vi "Initialize Debug Attribute.vi"(7 "Attribute.Debug in":refnum<class "Attribute.Debug.lvclass">, 11 "Behavior (Normal)":T1) -> (3 "Attribute.Debug out":refnum<class "Attribute.Debug.lvclass">)   [LabVIEW 2019, in "Debug.lvlib" / "Attribute.Debug.lvclass"]
uses:
  Attribute.Debug.lvclass
  DebugBehavior.ctl
  <vilib>/JKI/JKI SMO/smo.lvlibp/Definitions/def.SMO/Scope -- Enum.ctl
  Attribute.Debug.lvclass/Attribute.Debug.ctl
  <vilib>/JKI/JKI SMO/smo.lvlibp/Support/Attribute/Attribute.lvclass
  <vilib>/JKI/JKI SMO/smo.lvlibp/Definitions/def.SMO/def.SMO.lvclass
  C:/Program Files (x86)/National Instruments/LabVIEW 2019/vi.lib/JKI/JKI SMO/smo.lvlibp/Support/Attribute/Attribute.lvclass
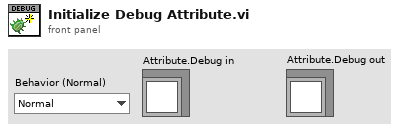
[diagram p1: front panel]
types:
  T1 = typedef "Debug.lvlib/Attribute.Debug.lvclass/DebugBehavior.ctl" = enum16{"Normal", "Debug"}
  T2 = typedef "smo.lvlibp/def.SMO.lvclass/Scope -- Enum.ctl" = enum16{"Public", "Protected", "Private"}
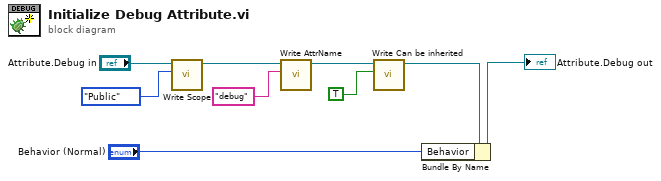
[diagram p0: block diagram]
diagram:
  n1 = call <vilib>:"Write Scope.vi"("Scope"=Scope_--_Enum."Public", "Attribute in"="Attribute.Debug in") -> ("Attribute out"=w7:refnum<class "Attribute.Debug.lvclass">)  [unwired: 9 in]
  n2 = call <vilib>:"Write AttrName.vi"("Attribute Name"="debug", "Attribute in"=w7) -> ("Attribute out"=w4:refnum<class "Attribute.Debug.lvclass">)  [unwired: 9 in]
  n3 = call <vilib>:"Write Can be inherited.vi"("Can be inherited"=TRUE, "Attribute in"=w4) -> ("Attribute out"=w3:refnum<class "Attribute.Debug.lvclass">)  [unwired: 8 in, 1 out]
  n4 = Bundle By Name(cluster=w3, "Behavior"="Behavior (Normal)") -> (→"Attribute.Debug out":refnum<class "Attribute.Debug.lvclass">)
